vi "BITOP-OR.vi"(0 "refnum in":refnum<vi>, 1 "Keys":string[](array[string]), 5 "Destination":string, 11 "error in":errorcluster) -> (4 "refnum out":refnum<vi>, 6 "Data":T1, 15 "error out":errorcluster)   [LabVIEW 2020]
uses:
  SubVIs/Controls/redis-data.ctl
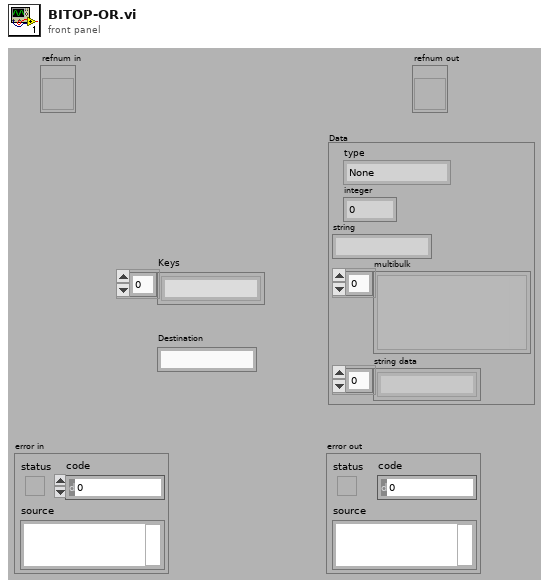
[diagram p1: front panel]
types:
  T1 = typedef "redis-data.ctl" = cluster{"type":enum16{"None", "Error", "Status", "Nil", "Integer", "String", "Multibulk"}, "integer":i64, "string":string, "multibulk":variant[], "string data":string[]}
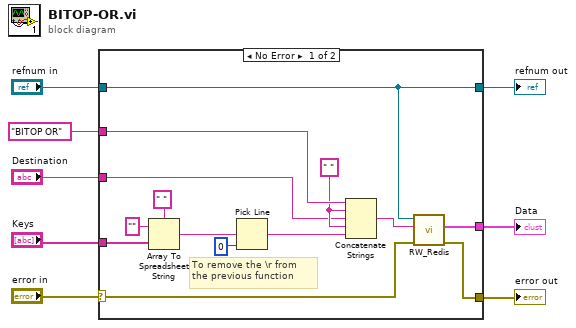
[diagram p0: block diagram]
diagram:
  n1 = case shown="No Error" "error in" {
    selector: "error in" -> [w15 w24]
    tunnel: "Keys" -> [w22 _]
    tunnel: "BITOP OR" -> [w12 _]
    tunnel: "refnum in" -> [w9 w23]
    tunnel: [w14 w24] -> w5
    tunnel: [w13 _] -> w1
    tunnel: "Destination" -> [w10 _]
    tunnel: [w9 w23] -> w2
    frame No Error {
      w11 = " "
      # "To remove the \\r from\nthe previous function"
      n2 = Array To Spreadsheet String(delimiter (Tab)=" ", array=w22, 3:"" ("format string")) -> (spreadsheet string=w18:string)
      n3 = Pick Line(multi-line string=w18, line index=0) -> (output string=w19:string)  [unwired: 1 in]
      n4 = Concatenate Strings(w12, w11, w10, w11, w19) -> (w16:string)
      n5 = call "RW_Redis.vi"("error in"=w15, "command"=w16, "refnum"=w9) -> ("error out"=w14:errorcluster, "Data"=w13:T1)  [unwired: 7 in]
    }
    frame Error {
    }
  }
  "error out" <- w5
  "refnum out" <- w2
  "Data" <- w1
